vi "7HP v2.0 external control - EnFlo_Specific.vi"(6 "Datalog file path (full)":path, 7 "COM port":refnum<visa-resource-name>, 8 "Log data stream":bool, 9 "Set data rate (Hz)":u8(ring)=14 items=["1", "2", "4", "5", "8", "10", "16", "20", "25", "32", "40", "50", "64", "80", "100", "125", "160", "200", "250", "320", "400", "500", "625", "800", "1000"], 10 "N samples":u32=1000, 11 "Command":T2="D") -> (0 "Error":errorcluster, 1 "Returned data rate (Hz)":u16, 2 "Serial number":sgl, 3 "Data out":T3[](array[typedef]) {"Time stamp" format="%<%.6X\n%x>T"}, 4 "Rendezvous out":bool)   [LabVIEW 2021]
doc: "7HP test and configuration software.\nVersion 2.0\nSurrey Sensors Ltd.\n11/2023"
uses:
  ctls/7HP_Cmd (USB).ctl
  ctls/7HP_Data cluster.ctl
  Globals/Meas_global.vi
panel:
  in  "COM port 2":refnum<visa-resource-name>
  in  "Main":T1(tab)
  out "Subsystems ok":bool[](array[boolean])
  out "Pressure sensor values in range":bool[](array[boolean])
  out "Pressure sensor temperatures in range":bool[](array[boolean])
  out "Pressure sensor EEPROM checksums ok":bool[](array[boolean])
  out "P_raw_Azero":sgl[](array[numeric])
  out "n":u16
  out "Auto zero progBar":u16(slide) caption="Collecting samples, please maintain dP = 0" scale=0.0..1000.0
  in  "EEPROM array 2":u16[](array[numeric])
  in  "EEPROM array":sgl[](array[numeric]) format="%#.3f"
  out "EEPROM checksum ok":bool
  out "EEPROM checksum":u16 format="%04x"
  out "received":bool
  out "sent":bool
  out "Processed outputs":sgl[](array[numeric]) format="%#.2f"
  out "Frame errors":u32
  out "Checksum errors":u32
  in  "Stop Data":bool
  out "Rel. humidity (%)":sgl format="%#.2f"
  out "T_board (°C)":sgl format="%#.2f"
  out "T_external (°C)":sgl format="%#.2f"
  out "P_atmos (mbar)":sgl format="%#.2f"
  out "Checksum ok":bool
  out "Gyration vector (° / s)":sgl[](array[numeric]) format="%#.3f"
  out "Acceleration vector (g)":sgl[](array[numeric]) format="%#.3f"
  out "Pressures":sgl[][](graph)
  out "Stream enabled":bool
  out "Pitch (°)":sgl format="%.2f"
  out "Roll (°)":sgl format="%.2f"
  # "Paul Nathan 01/2024"
  # "Pressure sensor 0 EEPROM checksum okay"
  # "Pressure sensor 0 value in range"
  # "Pressure sensor 1 EEPROM checksum okay"
  # "Pressure sensor 1 value in range"
  # "Pressure sensor 2 EEPROM checksum okay"
  # "Pressure sensor 2 value in range"
  # "Pressure sensor 3 EEPROM checksum okay"
  # "Pressure sensor 3 value in range"
  # "Pressure sensor 4 EEPROM checksum okay"
  # "Pressure sensor 4 value in range"
  # "Pressure sensor 5 EEPROM checksum okay"
  # "Pressure sensor 5 value in range"
  # "Pressure sensor 6 EEPROM checksum okay"
  # "Pressure sensor 6 value in range"
  # "Pressure sensor 0 temperature in range"
  # "Environmental sensor present"
  # "Pressure sensor 1 temperature in range"
  # "Inertial sensor present"
  # "Pressure sensor 2 temperature in range"
  # "Accelerometer self test pass"
  # "Pressure sensor 3 temperature in range"
  # "Gyroscope self test pass"
  # "Pressure sensor 4 temperature in range"
  # "External thermistor value in range"
  # "Pressure sensor 5 temperature in range"
  # "MCU EEPROM checksum ok"
  # "Pressure sensor 6 temperature in range"
  # "%"
  # "P0 raw auto-zero"
  # "P1 raw auto-zero"
  # "P2 raw auto-zero"
  # "P3 raw auto-zero"
  # "P4 raw auto-zero"
  # "P5 raw auto-zero"
  # "P6 raw auto-zero"
  # "Power-up defaults"
  # "P0 raw auto-zero"
  # "Data rate (Hz)"
  # "P1 raw auto-zero"
  # "TTL streaming"
  # "P2 raw auto-zero"
  # "USB streaming"
  # "P3 raw auto-zero"
  # "TTL stream contains full data"
  # "P4 raw auto-zero"
  # "Accelerometer range mode"
  # "P5 raw auto-zero"
  # "Gyroscope range mode"
  # "P6 raw auto-zero"
  # "IMU rate mode"
  # "Atmospheric pressure offset (Pa)"
  # "HW trigger edge polarity"
  # "External thermistor temperature offset (°C)"
  # "Serial number"
  # "TTL baud rate (bps)"
  # "Accelerometer vector magnitude scale factor"
  # "Gyroscope x component offset (deg / s)"
  # "Gyroscope y component offset (deg / s)"
  # "Gyroscope z component offset (deg / s)"
  # "||U|| (m/s)"
  # "Pitch (deg)"
  # "Yaw (deg)"
  # "U (m/s)"
  # "V (m/s)"
  # "W (m/s)"
  # "w_x"
  # "w_y"
  # "w_z"
  # "a_x"
  # "a_y"
  # "a_z"
  # "||U|| (m/s)"
  # "Pitch (deg)"
  # "Yaw (deg)"
  # "U (m/s)"
  # "V (m/s)"
  # "W (m/s)"
  # "w_x"
  # "w_y"
  # "w_z"
  # "a_x"
  # "a_y"
  # "a_z"
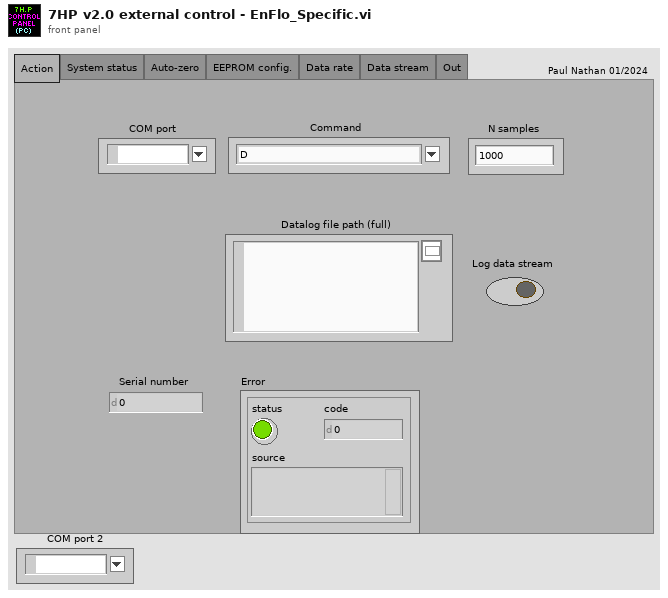
[diagram p1: front panel]
types:
  T1 = enum32{"Action", "System status", "Auto-zero", "EEPROM config.", "Data rate", "Data stream", "Out"}
  T2 = typedef "7HP_Cmd (USB).ctl" = string
  T3 = typedef "7HP_Data cluster.ctl" = cluster{"Time stamp":timestamp, "Pressures (Pa)":sgl[], "T_external (°C)":sgl, "P_atmos (mbar)":sgl, "T_board (°C)":sgl, "Rel. humidity (%)":sgl, "Acceleration vector (g)":sgl[], "Gyration vector (deg / s)":sgl[], "Processed outputs":sgl[]}
  T4 = enum16{"open", "replace", "create", "open or create", "replace or create", "replace or create with confirmation"}
  T5 = typedef "Rendezvous RefNum" = refnum<k1>
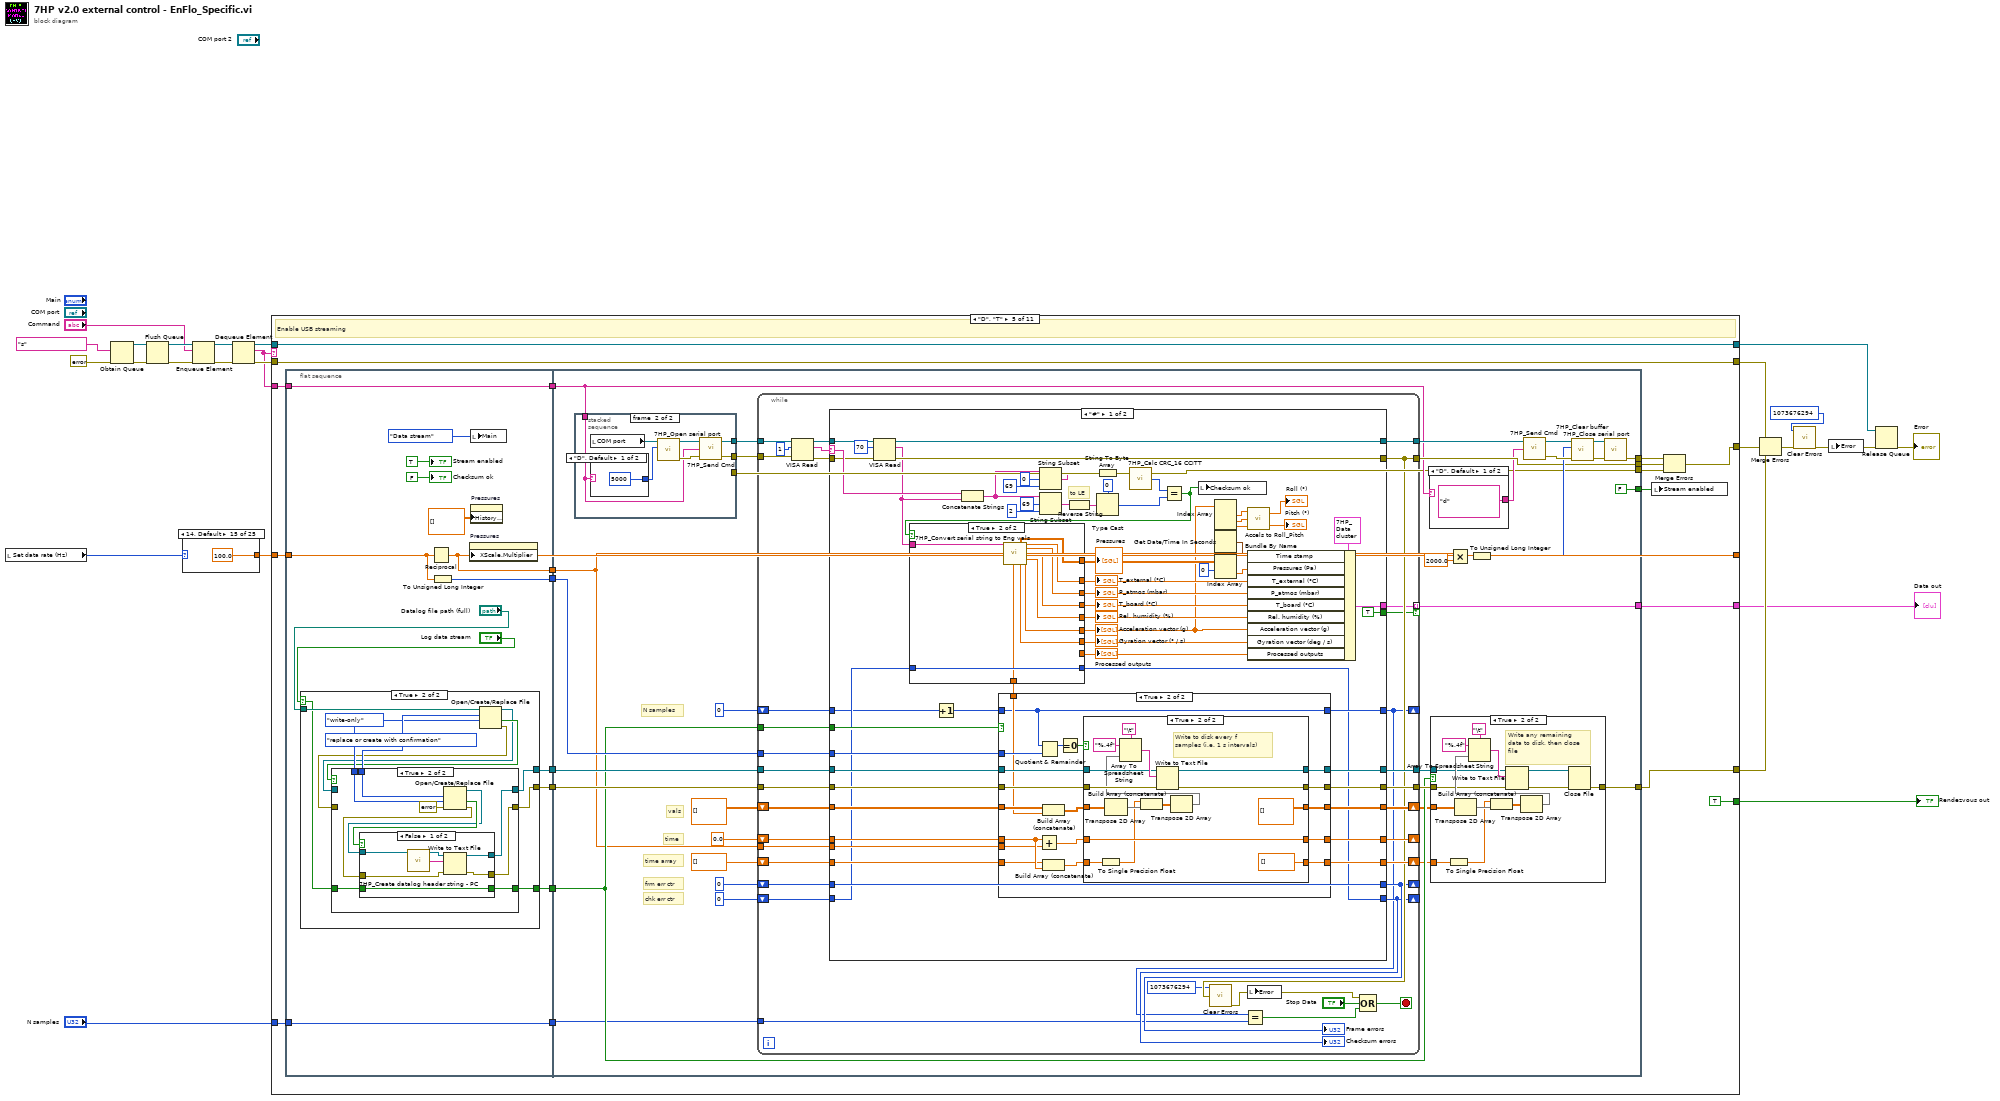
[diagram p0: block diagram]
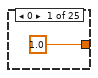
[diagram p2: hidden frame]
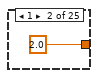
[diagram p3: hidden frame]
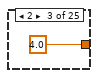
[diagram p4: hidden frame]
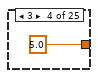
[diagram p5: hidden frame]
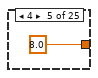
[diagram p6: hidden frame]
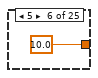
[diagram p7: hidden frame]
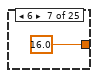
[diagram p8: hidden frame]
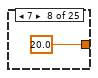
[diagram p9: hidden frame]
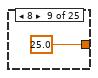
[diagram p10: hidden frame]
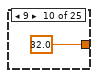
[diagram p11: hidden frame]
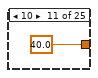
[diagram p12: hidden frame]
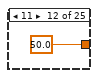
[diagram p13: hidden frame]
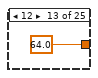
[diagram p14: hidden frame]
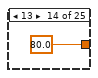
[diagram p15: hidden frame]
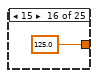
[diagram p16: hidden frame]
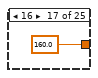
[diagram p17: hidden frame]
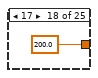
[diagram p18: hidden frame]
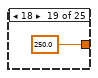
[diagram p19: hidden frame]
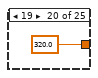
[diagram p20: hidden frame]
diagram:
  n1 = local read "Set data rate (Hz)"() -> (w4:u8)
  n2 = Obtain Queue(element data type=T2 "s" ("Combo Box"), error in (no error)=errorcluster {"status"=FALSE, "code"=0, "source"=""}) -> (queue out=w23:refnum<queue>, error out=w24:errorcluster)  [unwired: 3 in, 1 out]
  n3 = Flush Queue(queue=w23, error in (no error)=w24) -> (queue out=w19:refnum<queue>, error out=w20:errorcluster)  [unwired: 1 out]
  n4 = case shown="14, Default" w4 {
    tunnel: [1.0 2.0 4.0 5.0 8.0 10.0 16.0 20.0 25.0 32.0 40.0 50.0 64.0 80.0 100.0 125.0 160.0 200.0 250.0 320.0 400.0 500.0 625.0 800.0 1000.0] -> w5
    frame 0 {
    }
    frame 1 {
    }
    frame 2 {
    }
    frame 3 {
    }
    frame 4 {
    }
    frame 5 {
    }
    frame 6 {
    }
    frame 7 {
    }
    frame 8 {
    }
    frame 9 {
    }
    frame 10 {
    }
    frame 11 {
    }
    frame 12 {
    }
    frame 13 {
    }
    frame 14, Default {
    }
    frame 15 {
    }
    frame 16 {
    }
    frame 17 {
    }
    frame 18 {
    }
    frame 19 {
    }
    frame 20 {
    }
    frame 21 {
    }
    frame 22 {
    }
    frame 23 {
    }
    frame 24 {
    }
  }
  n5 = Enqueue Element(queue=w19, element="Command", error in (no error)=w20) -> (queue out=w18:refnum<queue>, error out=w17:errorcluster)  [unwired: 1 in, 1 out]
  n6 = Dequeue Element(queue=w18, error in (no error)=w17) -> (queue out=w15:refnum<queue>, element=w13:T2, error out=w14:errorcluster)  [unwired: 1 in, 1 out]
  n7 = case shown="\"D\", \"T\"" w13 {
    tunnel: [_ _ _ _ TRUE _ _ _ _ _ _] -> w1
    tunnel: w15 -> [w56 w95 w128 w190 w258 w547 w571 w627 w663 w685 w689]
    tunnel: [w56 w95 w128 w190 w258 w547 w571 w627 w663 w685 w689] -> w7
    tunnel: w14 -> [w55 w94 w127 w189 w257 w546 w572 w628 w662 w684 w688]
    tunnel: [w55 w94 w127 w189 w257 w546 w572 w628 w662 w684 w688] -> w12
    tunnel: w13 -> [w54 w93 w132 w196 w256 w549 w577 w633 w661 _ _]
    tunnel: [w52 w91 w130 w188 w244 w548 w570 w626 w659 errorcluster {"status"=FALSE, "code"=0, "source"=""} ("Error out") errorcluster {"status"=FALSE, "code"=0, "source"=""} ("Error out")] -> w11
    tunnel: [_ _ _ _ w254 _ _ _ _ _ _] -> w10
    tunnel: w5 -> [w51 w90 w129 w193 w247 w544 _ _ w658 w682 w686]
    tunnel: [w51 w90 w129 w193 w247 w544 w573 w629 w658 w682 w686] -> _
    tunnel: "N samples" -> [_ _ _ _ w242 _ _ _ _ _ _]
    tunnel: [_ _ _ _ w241 _ _ _ _ _ _] -> w2
    frame "S", "s" {
      # "Perform self-test and retrieve status bytes, Retrieve status bytes"
      n8 = flat-sequence {
        tunnel: w54 -> [w59]
        tunnel: [w59] -> w53
        tunnel: w53 -> [w65]
        tunnel: [w60] -> w52
        frame #0 {
          w58 = bool[] [] ("Pressure sensor EEPROM checksums ok")
          n9 = local write "Main"(T1."System status" ("Main")) -> ()
          "Pressure sensor EEPROM checksums ok" <- w58
          "Pressure sensor temperatures in range" <- w58
          "Pressure sensor values in range" <- w58
          "Subsystems ok" <- w58
        }
        frame #1 {
          w69 = 1 ("length (rest)")
          w77 = u8 0 ("byte count")
          n10 = local read "COM port"() -> (w66:refnum<visa-resource-name>)
          n11 = call "7HP_Open serial port.vi"("timeout (ms)"=u32 5000, "VISA resource name"=w66) -> ("Error out"=w87:errorcluster, "VISA resource name out"=w88:refnum<visa-resource-name>)  [unwired: 8 in]
          n12 = call "7HP_Send Cmd.vi"("Error In"=w87, "Operation"=w65, "Port"=w88) -> ("Error Out"=w85:errorcluster, "Port out"=w86:refnum<visa-resource-name>)  [unwired: 1 in]
          n13 = VISA Read(VISA resource name=w86, byte count=u32 4, error in (no error)=w85) -> (VISA resource name out=w83:refnum<visa-resource-name>, read buffer=w72:string, error out=w82:errorcluster)  [unwired: 1 out]
          n14 = call "7HP_Close serial port.vi"("Error in"=w82, "VISA resource name"=w83) -> ("Error out"=w60:errorcluster)  [unwired: 9 in]
          n15 = String Subset(string=w72, offset (0)=0, length (rest)=w69) -> (substring=w81:string)
          n16 = String Subset(string=w72, offset (0)=1, length (rest)=w69) -> (substring=w80:string)
          n17 = String Subset(string=w72, offset (0)=2 ("length (rest)"), length (rest)=w69) -> (substring=w79:string)
          n18 = String Subset(string=w72, offset (0)=3, length (rest)=w69) -> (substring=w78:string)
          n19 = Type Cast(type=w77, x=w81) -> (*(type *) &x=w76:u8)
          n20 = Type Cast(type=w77, x=w80) -> (*(type *) &x=w75:u8)
          n21 = Type Cast(type=w77, x=w79) -> (*(type *) &x=w74:u8)
          n22 = Type Cast(type=w77, x=w78) -> (*(type *) &x=w73:u8)
          n23 = Number To Boolean Array(number=w76) -> (Boolean array=w64:bool[])
          n24 = Number To Boolean Array(number=w75) -> (Boolean array=w63:bool[])
          n25 = Number To Boolean Array(number=w74) -> (Boolean array=w62:bool[])
          n26 = Number To Boolean Array(number=w73) -> (Boolean array=w61:bool[])
          n27 = local write "Pressure sensor EEPROM checksums ok"(w64) -> ()
          n28 = local write "Pressure sensor temperatures in range"(w63) -> ()
          n29 = local write "Pressure sensor values in range"(w62) -> ()
          n30 = local write "Subsystems ok"(w61) -> ()
        }
      }
    }
    frame "Z", "z" {
      # "Perform permanent auto-zero (write values to EEPROM), Perform temporary auto-zero"
      n31 = flat-sequence {
        tunnel: w93 -> [w99]
        tunnel: [w99] -> w92
        tunnel: w92 -> [w106]
        tunnel: [w102] -> w91
        frame #0 {
          n32 = local write "Main"(T1."Auto-zero" ("Main")) -> ()
          "P_raw_Azero" <- sgl[] [] ("P_raw_Azero")
          "Auto zero progBar" <- u16 0 ("Collecting samples, please maintain dP = 0")
        }
        frame #1 {
          n33 = local read "COM port"() -> (w107:refnum<visa-resource-name>)
          n34 = call "7HP_Open serial port.vi"("timeout (ms)"=u32 16000, "VISA resource name"=w107) -> ("Error out"=w113:errorcluster, "VISA resource name out"=w114:refnum<visa-resource-name>)  [unwired: 8 in]
          n35 = call "7HP_Send Cmd.vi"("Error In"=w113, "Operation"=w106, "Port"=w114) -> ("Error Out"=w111:errorcluster, "Port out"=w112:refnum<visa-resource-name>)  [unwired: 1 in]
          n36 = VISA Read(VISA resource name=w112, byte count=u32 28, error in (no error)=w111) -> (VISA resource name out=w109:refnum<visa-resource-name>, read buffer=w103:string, error out=w108:errorcluster)  [unwired: 1 out]
          n37 = for {
            N: 100 -> [_]
            shift-right: [w116] -> _
            shift-left: u16 0 -> [w117]
            n38 = Increment(x=w117) -> (x+1=w116:u16)
            "n" <- w116
            n39 = Wait (ms)(milliseconds to wait=u32 100) -> ()  [unwired: 1 out]
            n40 = local write "Auto zero progBar"(w116) -> ()
          }
          n41 = for {
            N: 7 -> [_]
            tunnel: [w120] -> w105 mode=indexing
            tunnel: w103 -> [w119]
            i -> [w126]
            w124 = 4 ("x")
            # "to BE"
            n42 = Multiply(x=w124, y=w126) -> (x*y=w125:i32)
            n43 = String Subset(string=w119, offset (0)=w125, length (rest)=w124) -> (substring=w123:string)
            n44 = Reverse String(1:w123) -> (0:w122:string)
            n45 = Type Cast(type=sgl 0.0 ("byte count"), x=w122) -> (*(type *) &x=w120:sgl)
          }
          n46 = call "7HP_Close serial port.vi"("Error in"=w108, "VISA resource name"=w109) -> ("Error out"=w102:errorcluster)  [unwired: 9 in]
          n47 = local write "P_raw_Azero"(w105) -> ()
        }
      }
    }
    frame "R" {
      # "Read all EEPROM values"
      n48 = flat-sequence {
        tunnel: w132 -> [w138]
        tunnel: [w138] -> w131
        tunnel: w131 -> [w170]
        tunnel: [w168] -> w130
        frame #0 {
          n49 = local write "EEPROM checksum ok"(FALSE ("Chk ok")) -> ()
          n50 = local write "EEPROM checksum"(u16 0 ("EEPROM checksum")) -> ()
          n51 = local write "EEPROM array"(sgl[] [] ("EEPROM array")) -> ()
          n52 = local write "EEPROM array 2"(u16[] [] ("EEPROM array 2")) -> ()
          n53 = local write "Main"(T1."EEPROM config." ("Main")) -> ()
        }
        frame #1 {
          # "to BE"
          # "to BE"
          n54 = local read "COM port"() -> (w171:refnum<visa-resource-name>)
          n55 = call "7HP_Open serial port.vi"("timeout (ms)"=u32 5000, "VISA resource name"=w171) -> ("Error out"=w177:errorcluster, "VISA resource name out"=w178:refnum<visa-resource-name>)  [unwired: 8 in]
          n56 = call "7HP_Send Cmd.vi"("Error In"=w177, "Operation"=w170, "Port"=w178) -> ("Error Out"=w175:errorcluster, "Port out"=w176:refnum<visa-resource-name>)  [unwired: 1 in]
          n57 = VISA Read(VISA resource name=w176, byte count=u32 71, error in (no error)=w175) -> (VISA resource name out=w173:refnum<visa-resource-name>, read buffer=w144:string, error out=w172:errorcluster)  [unwired: 1 out]
          n58 = call "7HP_Close serial port.vi"("Error in"=w172, "VISA resource name"=w173) -> ("Error out"=w168:errorcluster)  [unwired: 9 in]
          n59 = String Subset(string=w144, offset (0)=0, length (rest)=60 ("length (rest)")) -> (substring=w167:string)
          n60 = String Subset(string=w144, offset (0)=60, length (rest)=2 ("length (rest)")) -> (substring=w158:string)
          n61 = String Subset(string=w144, offset (0)=62, length (rest)=7 ("length (rest)")) -> (substring=w153:string)
          n62 = String Subset(string=w144, offset (0)=69, length (rest)=2 ("length (rest)")) -> (substring=w145:string)
          n63 = String Subset(string=w144, offset (0)=0, length (rest)=69 ("length (rest)")) -> (substring=w141:string)
          n64 = for {
            N: 15 -> [_]
            tunnel: [w183] -> w139 mode=indexing
            tunnel: w167 -> [w182]
            i -> [w187]
            w185 = 4 ("x")
            # "to BE"
            n65 = Multiply(x=w185, y=w187) -> (x*y=w186:i32)
            n66 = String Subset(string=w182, offset (0)=w186, length (rest)=w185) -> (substring=w181:string)
            n67 = Reverse String(1:w181) -> (0:w180:string)
            n68 = Type Cast(type=sgl 0.0 ("byte count"), x=w180) -> (*(type *) &x=w183:sgl)
          }
          n69 = Reverse String(1:w158) -> (0:w164:string)
          n70 = Reverse String(1:w145) -> (0:w149:string)
          n71 = String To Byte Array(string=w141) -> (unsigned byte array=w152:u8[])
          n72 = call "7HP_Calc CRC_16 CCITT.vi"("Data bytes"=w152) -> ("CRC_16-CCITT"=w151:u16)  [unwired: 1 in]
          n73 = Type Cast(type=u16 0 ("byte count"), x=w164) -> (*(type *) &x=w157:u16)
          n74 = Type Cast(type=u16 0 ("byte count"), x=w149) -> (*(type *) &x=w140:u16)
          n75 = String To Byte Array(string=w153) -> (unsigned byte array=w156:u8[])
          n76 = To Unsigned Word Integer(number=w156) -> (unsigned 16bit integer=w154:u16[])
          n77 = Equal?(x=w140, y=w151) -> (x = y?=w150:bool)
          n78 = Build Array (concatenate)(w157, w154) -> (w155:u16[])
          n79 = local write "EEPROM checksum ok"(w150) -> ()
          n80 = local write "EEPROM array"(w139) -> ()
          n81 = local write "EEPROM array 2"(w155) -> ()
          n82 = local write "EEPROM checksum"(w140) -> ()
        }
      }
    }
    frame "W" {
      # "Write all EEPROM values (including new checksum)"
      n83 = flat-sequence {
        tunnel: w196 -> [w206]
        tunnel: [w206] -> w195
        tunnel: ["EEPROM array"] -> w194
        tunnel: [w200] -> w192
        tunnel: [w201] -> w191
        tunnel: w195 -> [w228]
        tunnel: w194 -> [w223]
        tunnel: [w222] -> w188
        tunnel: w192 -> [w214]
        tunnel: w191 -> [w212]
        frame #0 {
          n84 = local write "Main"(T1."EEPROM config." ("Main")) -> ()
          n85 = Split 1D Array(array="EEPROM array 2", index=1) -> (first subarray=w203:u16[], second subarray=w202:u16[])
          n86 = Index Array(array=w203, index=0) -> (element=w200:u16)
          n87 = To Unsigned Byte Integer(number=w202) -> (unsigned 8bit integer=w201:u8[])
        }
        frame #1 {
          # "to LE"
          # "to LE"
          n88 = local read "COM port"() -> (w229:refnum<visa-resource-name>)
          n89 = for {
            N: 15 -> [_]
            tunnel: w223 -> [w235] mode=indexing
            shift-right: [w236] -> w218
            shift-left: "" -> [w237]
            # "to LE"
            n90 = Type Cast(type="", x=w235) -> (*(type *) &x=w234:string)
            n91 = Reverse String(1:w234) -> (0:w233:string)
            n92 = Concatenate Strings(w237, w233) -> (w236:string)
          }
          n93 = Type Cast(type="", x=w214) -> (*(type *) &x=w216:string)
          n94 = Reverse String(1:w216) -> (0:w213:string)
          n95 = Byte Array To String(unsigned byte array=w212) -> (string=w211:string)
          n96 = call "7HP_Open serial port.vi"("timeout (ms)"=u32 5000, "VISA resource name"=w229) -> ("Error out"=w230:errorcluster, "VISA resource name out"=w231:refnum<visa-resource-name>)  [unwired: 8 in]
          n97 = Concatenate Strings(w218, w213, w211) -> (w217:string)
          n98 = String To Byte Array(string=w217) -> (unsigned byte array=w210:u8[])
          n99 = call "7HP_Calc CRC_16 CCITT.vi"("Data bytes"=w210) -> ("CRC_16-CCITT"=w209:u16)  [unwired: 1 in]
          "EEPROM checksum" <- w209
          n100 = Type Cast(type="", x=w209) -> (*(type *) &x=w208:string)
          n101 = Reverse String(1:w208) -> (0:w207:string)
          n102 = Concatenate Strings(w217, w207) -> (w221:string)
          n103 = call "7HP_Send Cmd + Data.vi"("Error In"=w230, "Data"=w221, "Operation"=w228, "Port"=w231) -> ("Error Out"=w219:errorcluster, "Port out"=w220:refnum<visa-resource-name>)  [unwired: 1 in]
          n104 = call "7HP_Close serial port.vi"("Error in"=w219, "VISA resource name"=w220) -> ("Error out"=w222:errorcluster)  [unwired: 9 in]
          "EEPROM checksum ok" <- TRUE ("Chk ok")
        }
      }
    }
    frame "D", "T" {
      # "Enable USB streaming"
      n105 = flat-sequence {
        tunnel: w256 -> [w272]
        tunnel: [w272] -> w255
        tunnel: [w269] -> w253
        tunnel: [w268] -> w252
        tunnel: [w267] -> w251
        tunnel: w247 -> [w262]
        tunnel: [w261] -> w250
        tunnel: [w263] -> w249
        tunnel: [w260] -> w243
        tunnel: w242 -> [w260]
        tunnel: w255 -> [w314]
        tunnel: [w344] -> w245
        tunnel: [w343] -> w254
        tunnel: w253 -> [w340]
        tunnel: w252 -> [w339]
        tunnel: w251 -> [w341]
        tunnel: w250 -> [w323]
        tunnel: w249 -> [w333]
        tunnel: [FALSE] -> w248
        tunnel: [w318] -> w246
        tunnel: w243 -> [w315]
        tunnel: [w312] -> w241
        tunnel: [w311] -> w240
        frame #0 {
          n106 = case shown="True" "Log data stream" {
            selector: "Log data stream" -> [w273 w276]
            tunnel: "Datalog file path (full)" -> [_ w285]
            tunnel: [refnum<file> refnum ("refnum out") w282] -> w269
            tunnel: [errorcluster {"status"=FALSE, "code"=0, "source"=""} ("error out") w281] -> w268
            tunnel: [w273 w277] -> w263
            frame False {
            }
            frame True {
              w283 = enum16{"read/write", "read-only", "write-only"}."write-only" ("access (0:read/write)")
              w284 = T4."replace or create with confirmation" ("operation (0:open)")
              n107 = Open/Create/Replace File(file path (use dialog)=w285, operation (0:open)=w284, access (0:read/write)=w283) -> (refnum out=w278:refnum<file>, cancelled=w280:bool, error out=w279:errorcluster)  [unwired: 3 in]
              n108 = case shown="True" w280 {
                tunnel: w284 -> [_ w301]
                tunnel: w283 -> [_ w300]
                tunnel: w279 -> [w289 _]
                tunnel: [w287 w295] -> w282
                tunnel: [w288 w296] -> w281
                tunnel: w278 -> [w290 _]
                tunnel: [w286 w293] -> w277
                tunnel: w276 -> [w286 w292]
                frame False {
                  n109 = call "7HP_Create datalog header string - PC.vi"() -> ("Datalog header string"=w291:string)  [unwired: 1 in]
                  n110 = Write to Text File(file (use dialog)=w290, text=w291, error in=w289) -> (refnum out=w287:refnum<file>, error out=w288:errorcluster)  [unwired: 1 in, 1 out]
                }
                frame True {
                  n111 = Open/Create/Replace File(error in=errorcluster {"status"=FALSE, "code"=0, "source"=""}, operation (0:open)=w301, access (0:read/write)=w300) -> (refnum out=w298:refnum<file>, cancelled=w299:bool, error out=w297:errorcluster)  [unwired: 3 in]
                  n112 = case shown="False" w299 {
                    tunnel: w298 -> [w306 _]
                    tunnel: w297 -> [w305 _]
                    tunnel: [w304 errorcluster {"status"=FALSE, "code"=0, "source"=""} ("error out")] -> w296
                    tunnel: [w303 refnum<file> refnum ("t")] -> w295
                    tunnel: [w302 w308] -> w293
                    tunnel: w292 -> [w302 _]
                    frame False {
                      n113 = call "7HP_Create datalog header string - PC.vi"() -> ("Datalog header string"=w307:string)  [unwired: 1 in]
                      n114 = Write to Text File(file (use dialog)=w306, text=w307, error in=w305) -> (refnum out=w303:refnum<file>, error out=w304:errorcluster)  [unwired: 1 in, 1 out]
                    }
                    frame True {
                      w308 = FALSE ("Log data stream")
                      n115 = local write "Log data stream"(w308) -> ()
                    }
                  }
                }
              }
            }
          }
          n116 = Reciprocal(x=w262) -> (1/x=w261:dbl)
          n117 = To Unsigned Long Integer(number=w262) -> (unsigned 32bit integer=w267:u32)
          n118 = property on="Pressures" class="WFChart (strict)"("XScale.Multiplier"=w261) -> ()  [unwired: 2 in, 2 out]
          n119 = local write "Main"(T1."Data stream" ("Main")) -> ()
          n120 = property on="Pressures" class="WFChart (strict)"("History Data"=sgl[][] []) -> ()  [unwired: 2 in, 2 out]
          "Checksum ok" <- FALSE ("Checksum ok")
          "Stream enabled" <- TRUE ("Stream enabled")
        }
        frame #1 {
          # "N samples"
          # "chk err ctr"
          # "frm err ctr"
          # "vals"
          # "time"
          # "time array"
          n121 = stacked-sequence {
            tunnel: [_ w352] -> w332
            tunnel: [_ w350] -> w331
            tunnel: w314 -> [_ w348]
            tunnel: [w345 _] -> w311
            frame #0 {
              # "Wait here until all acq. devs. are ready."
              n122 = global read "Meas_global.vi" "Acquisition Rendezvous"() -> (w347:T5)
              n123 = call <vilib>:"Wait at Rendezvous.vi"("ms timeout (-1)"=60000, "rendezvous"=w347) -> ("error out"=w345:errorcluster)  [unwired: 3 in, 2 out]
            }
            frame #1 {
              n124 = local read "COM port"() -> (w354:refnum<visa-resource-name>)
              n125 = case shown="\"D\", Default" w348 {
                tunnel: [u32 5000 ("timeout (ms)") u32 15000 ("timeout (ms)")] -> w349
                frame "D", Default {
                }
                frame "T" {
                }
              }
              n126 = call "7HP_Open serial port.vi"("timeout (ms)"=w349, "VISA resource name"=w354) -> ("Error out"=w351:errorcluster, "VISA resource name out"=w353:refnum<visa-resource-name>)  [unwired: 8 in]
              n127 = call "7HP_Send Cmd.vi"("Error In"=w351, "Operation"=w348, "Port"=w353) -> ("Error Out"=w350:errorcluster, "Port out"=w352:refnum<visa-resource-name>)  [unwired: 1 in]
            }
          }
          n128 = while {
            tunnel: [w370] -> w318
            tunnel: w332 -> [w372]
            tunnel: [w389] -> w330
            shift-right: [w363] -> _
            shift-left: u32 0 -> [w386]
            tunnel: w341 -> [w385]
            tunnel: w340 -> [w384]
            tunnel: w339 -> [w383]
            tunnel: [w382] -> w338
            tunnel: [w381] -> w337
            shift-right: [w380] -> w320
            shift-left: sgl[][] [] -> [w379]
            shift-right: [w376] -> _
            shift-left: 0.0 ("Numeric") -> [w378]
            tunnel: w323 -> [w377]
            shift-right: [w374] -> w319
            shift-left: dbl[] [] -> [w375]
            tunnel: w333 -> [w373]
            tunnel: w331 -> [w371]
            shift-right: [w365] -> _
            shift-left: u32 0 -> [w367]
            shift-right: [w364] -> _
            shift-left: u32 0 -> [w366]
            tunnel: w315 -> [w362]
            tunnel: [w360] -> w312 mode=indexing if=w359
            stop <- w387 stop-if-true
            n129 = VISA Read(VISA resource name=w372, byte count=u32 1, error in (no error)=w371) -> (VISA resource name out=w391:refnum<visa-resource-name>, read buffer=w392:string, error out=w390:errorcluster)  [unwired: 1 out]
            n130 = case shown="\"#\"" w392 {
              selector: w392 -> [w435 _]
              tunnel: w391 -> [w421 w527]
              tunnel: [w451 w528] -> w370
              tunnel: w390 -> [w420 w528]
              tunnel: [w452 w527] -> w389
              tunnel: w386 -> [w414 w526]
              tunnel: [w450 w526] -> w363
              tunnel: w385 -> [w449 _]
              tunnel: w384 -> [w448 w525]
              tunnel: w383 -> [w447 w524]
              tunnel: [w446 w524] -> w382
              tunnel: [w445 w525] -> w381
              tunnel: [w444 w523] -> w380
              tunnel: w379 -> [w443 w523]
              tunnel: w378 -> [w442 w522]
              tunnel: w377 -> [w441 _]
              tunnel: [w440 w522] -> w376
              tunnel: w375 -> [w439 w521]
              tunnel: [w438 w521] -> w374
              tunnel: w373 -> [w437 _]
              tunnel: w367 -> [w436 w520]
              tunnel: w366 -> [w416 w519]
              tunnel: [w436 w518] -> w365
              tunnel: [w415 w519] -> w364
              tunnel: [w409 _] -> w360
              tunnel: [TRUE FALSE] -> w359
              frame "#" {
                # "to LE"
                n131 = VISA Read(VISA resource name=w421, byte count=u32 70, error in (no error)=w420) -> (VISA resource name out=w452:refnum<visa-resource-name>, read buffer=w419:string, error out=w451:errorcluster)  [unwired: 1 out]
                n132 = Increment(x=w414) -> (x+1=w413:u32)
                n133 = Concatenate Strings(w435, w419) -> (w423:string)
                n134 = String Subset(string=w423, offset (0)=0, length (rest)=69 ("length (rest)")) -> (substring=w422:string)
                n135 = String Subset(string=w423, offset (0)=69, length (rest)=2 ("length (rest)")) -> (substring=w429:string)
                n136 = Reverse String(1:w429) -> (0:w428:string)
                n137 = String To Byte Array(string=w422) -> (unsigned byte array=w433:u8[])
                n138 = Type Cast(type=u16 0 ("length (rest)"), x=w428) -> (*(type *) &x=w427:u16)
                n139 = call "7HP_Calc CRC_16 CCITT.vi"("Data bytes"=w433) -> ("CRC_16-CCITT"=w426:u16)  [unwired: 1 in]
                n140 = Equal?(x=w426, y=w427) -> (x = y?=w417:bool)
                n141 = case shown="True" w417 {
                  tunnel: w419 -> [_ w470]
                  tunnel: [w459 w469] -> w411
                  tunnel: [w455 w468] -> w405
                  tunnel: [w455 w467] -> w404
                  tunnel: [w455 w466] -> w403
                  tunnel: [w455 w465] -> w402
                  tunnel: [w454 w464] -> w394
                  tunnel: [w454 w463] -> w401
                  tunnel: [w456 w461] -> w418
                  tunnel: w416 -> [w458 w462]
                  tunnel: [w457 w462] -> w415
                  tunnel: [sgl[] [nan, nan, nan, nan, nan, nan] _] -> w400
                  frame False {
                    w460 = sgl[] [nan, nan, nan, nan, nan, nan, nan]
                    w455 = sgl nan
                    w454 = sgl[] [nan, nan, nan]
                    n142 = Increment(x=w458) -> (x+1=w457:u32)
                    n143 = Build Array (concatenate)(w460, w455, w455, w455, w455, w454, w454) -> (w456:sgl[])
                    n144 = Build Array(w460) -> (w459:sgl[][])
                  }
                  frame True {
                    n145 = call "7HP_Convert serial string to Eng vals.vi"("Serial buffer string (excluding FrameChar)"=w470) -> ("All vals"=w461:sgl[], "Pressures"=w469:sgl[][], "Gyration vector (deg / s)"=w463:sgl[], "External thermistor temperature (deg C)"=w468:sgl, "Atmospheric pressure (mbar)"=w467:sgl, "Env. sensor die temperature (deg C)"=w466:sgl, "Relative humidity (%)"=w465:sgl, "Acceleration vector (g)"=w464:sgl[])  [unwired: 11 in]
                  }
                }
                "Pressures" <- w411
                "Acceleration vector (g)" <- w394
                "Gyration vector (° / s)" <- w401
                "P_atmos (mbar)" <- w404
                "T_external (°C)" <- w405
                "T_board (°C)" <- w403
                "Rel. humidity (%)" <- w402
                "Processed outputs" <- w400
                n146 = case shown="True" w437 {
                  tunnel: w413 -> [w476 w477]
                  tunnel: [w476 w477] -> w450
                  tunnel: w449 -> [_ w495]
                  tunnel: w418 -> [_ w481]
                  tunnel: w448 -> [w474 w492]
                  tunnel: w447 -> [w475 w491]
                  tunnel: [w475 w490] -> w446
                  tunnel: [w474 w489] -> w445
                  tunnel: w443 -> [w473 w482]
                  tunnel: [w473 w488] -> w444
                  tunnel: w442 -> [w472 w485]
                  tunnel: w441 -> [_ w484]
                  tunnel: [w472 w487] -> w440
                  tunnel: w439 -> [w471 w483]
                  tunnel: [w471 w486] -> w438
                  frame False {
                  }
                  frame True {
                    n147 = Add(x=w485, y=w484) -> (x+y=w480:dbl)
                    n148 = Quotient & Remainder(x=w477, y=w495) -> (x-y*floor(x/y)=w494:u32)  [unwired: 1 out]
                    n149 = Build Array (concatenate)(w482, w481) -> (w478:sgl[][])
                    n150 = Build Array (concatenate)(w483, w485) -> (w479:dbl[])
                    n151 = Equal To 0?(x=w494) -> (x = 0?=w493:bool)
                    n152 = case shown="True" w493 {
                      tunnel: w492 -> [w499 w513]
                      tunnel: w491 -> [w500 w512]
                      tunnel: [w500 w511] -> w490
                      tunnel: [w499 w510] -> w489
                      tunnel: w478 -> [w497 w505]
                      tunnel: [w497 sgl[][] []] -> w488
                      tunnel: w480 -> [w498 w508]
                      tunnel: [w498 w508] -> w487
                      tunnel: w479 -> [w496 w507]
                      tunnel: [w496 dbl[] []] -> w486
                      frame False {
                      }
                      frame True {
                        # "Write to disk every f samples (i.e. 1 s intervals)"
                        n153 = To Single Precision Float(number=w507) -> (single precision float=w501:sgl[])
                        n154 = Transpose 2D Array(2D array=w505) -> (transposed array=w504:sgl[][])
                        n155 = Build Array (concatenate)(w501, w504) -> (w503:sgl[][])
                        n156 = Transpose 2D Array(2D array=w503) -> (transposed array=w502:sgl[][])
                        n157 = Array To Spreadsheet String(delimiter (Tab)="\t", array=w502, 3:"%.4f" ("format string")) -> (spreadsheet string=w516:string)
                        n158 = Write to Text File(file (use dialog)=w513, text=w516, error in=w512) -> (refnum out=w510:refnum<file>, error out=w511:errorcluster)  [unwired: 1 in, 1 out]
                      }
                    }
                  }
                }
                n159 = local write "Checksum ok"(w417) -> ()
                n160 = Index Array(array=w394) -> (element #1=w399:sgl, element #2=w398:sgl, element #3=w397:sgl)  [unwired: 3 in]
                n161 = Get Date/Time In Seconds() -> (seconds since 1Jan1904=w407:timestamp)
                n162 = Index Array(array=w411, index (row)=0) -> (element=w406:sgl[])  [unwired: 1 in]
                n163 = call "Accels to Roll_Pitch.vi"("az"=w397, "ay"=w398, "ax"=w399) -> ("Pitch (deg)"=→"Pitch (°)":sgl, "Roll (deg)"=→"Roll (°)":sgl)
                n164 = Bundle By Name(cluster=T3 {"Time stamp"=timestamp(0 s since 1904-01-01), "Pressures (Pa)"=[], "T_external (°C)"=0.0, "P_atmos (mbar)"=0.0, "T_board (°C)"=0.0, "Rel. humidity (%)"=0.0, "Acceleration vector (g)"=[], "Gyration vector (deg / s)"=[], "Processed outputs"=[]} ("Data cluster 7HP"), "Time stamp"=w407, "Pressures (Pa)"=w406, "T_external (°C)"=w405, "P_atmos (mbar)"=w404, "T_board (°C)"=w403, "Rel. humidity (%)"=w402, "Acceleration vector (g)"=w394, "Gyration vector (deg / s)"=w401, "Processed outputs"=w400) -> (w409:T3)
              }
              frame Default {
                # "Frame error"
                n165 = Increment(x=w520) -> (x+1=w518:u32)
              }
            }
            "Checksum errors" <- w364
            "Frame errors" <- w365
            n166 = call <vilib>:"Clear Errors.vi"("error in (no error)"=w370, "specific error code to clear (0: all)"=1073676294) -> ("error out"=w369:errorcluster)  [unwired: 4 in, 1 out]
            n167 = Equal?(x=w363, y=w362) -> (x = y?=w361:bool)
            n168 = local write "Error"(w369) -> ()
            n169 = Compound Arithmetic op=OR(w369, "Stop Data", w361) -> (w387:bool)
          }
          n170 = case shown="\"D\", Default" w314 {
            tunnel: [T2 "d" ("Combo Box") T2 "t" ("Combo Box")] -> w313
            frame "D", Default {
            }
            frame "T" {
            }
          }
          n171 = case shown="True" w333 {
            tunnel: [w529 w543] -> w343
            tunnel: w338 -> [w529 w535]
            tunnel: w337 -> [_ w536]
            tunnel: w320 -> [_ w534]
            tunnel: w319 -> [_ w533]
            frame False {
            }
            frame True {
              # "Write any remaining data to disk, then close file"
              n172 = To Single Precision Float(number=w533) -> (single precision float=w530:sgl[])
              n173 = Transpose 2D Array(2D array=w534) -> (transposed array=w540:sgl[][])
              n174 = Build Array (concatenate)(w530, w540) -> (w541:sgl[][])
              n175 = Transpose 2D Array(2D array=w541) -> (transposed array=w542:sgl[][])
              n176 = Array To Spreadsheet String(delimiter (Tab)="\t", array=w542, 3:"%.4f" ("format string")) -> (spreadsheet string=w537:string)
              n177 = Write to Text File(file (use dialog)=w536, text=w537, error in=w535) -> (refnum out=w532:refnum<file>, error out=w531:errorcluster)  [unwired: 1 in, 1 out]
              n178 = Close File(refnum=w532, error in=w531) -> (error out=w543:errorcluster)  [unwired: 1 out]
            }
          }
          n179 = Multiply(x=w323, y=2000.0) -> (x*y=w324:dbl)
          n180 = To Unsigned Long Integer(number=w324) -> (unsigned 32bit integer=w321:u32)
          n181 = call "7HP_Send Cmd.vi"("Operation"=w313, "Port"=w330) -> ("Error Out"=w327:errorcluster, "Port out"=w328:refnum<visa-resource-name>)  [unwired: 2 in]
          n182 = call "7HP_Clear buffer.vi"("Error in"=w327, "dt for timeout (ms)"=w321, "VISA resource name in"=w328) -> ("Error out"=w325:errorcluster, "VISA resource name out"=w326:refnum<visa-resource-name>)  [unwired: 3 in]
          n183 = call "7HP_Close serial port.vi"("Error in"=w325, "VISA resource name"=w326) -> ("Error out"=w344:errorcluster)  [unwired: 9 in]
        }
      }
      n184 = local write "Stream enabled"(w248) -> ()
      n185 = Merge Errors(w245, w246, w240) -> (w244:errorcluster)
    }
    frame "d", "t" {
      # "Disable USB streaming"
      n186 = flat-sequence {
        tunnel: [w557] -> w550
        tunnel: w549 -> [w557]
        tunnel: w544 -> [w556]
        tunnel: [w551] -> w545
        tunnel: w550 -> [w565]
        tunnel: [w564] -> w548
        tunnel: w545 -> [w559]
        frame #0 {
          n187 = Reciprocal(x=w556) -> (1/x=w555:dbl)
          n188 = disable-structure shown="Disabled" {
            frame Disabled {
              n189 = local write "Main"(T1."Data stream" ("Main")) -> ()
            }
            frame Enabled {
            }
          }
          n190 = To Single Precision Float(number=w555) -> (single precision float=w552:sgl)
          n191 = Multiply(x=w552, y=sgl 2000.0) -> (x*y=w553:sgl)
          n192 = To Unsigned Long Integer(number=w553) -> (unsigned 32bit integer=w551:u32)
        }
        frame #1 {
          n193 = local read "COM port"() -> (w566:refnum<visa-resource-name>)
          n194 = call "7HP_Open serial port.vi"("timeout (ms)"=u32 5000, "VISA resource name"=w566) -> ("Error out"=w567:errorcluster, "VISA resource name out"=w568:refnum<visa-resource-name>)  [unwired: 8 in]
          n195 = call "7HP_Send Cmd.vi"("Error In"=w567, "Operation"=w565, "Port"=w568) -> ("Error Out"=w563:errorcluster, "Port out"=w561:refnum<visa-resource-name>)  [unwired: 1 in]
          n196 = call "7HP_Clear buffer.vi"("Error in"=w563, "dt for timeout (ms)"=w559, "VISA resource name in"=w561) -> ("Error out"=w562:errorcluster, "VISA resource name out"=w560:refnum<visa-resource-name>)  [unwired: 3 in]
          n197 = call "7HP_Close serial port.vi"("Error in"=w562, "VISA resource name"=w560) -> ("Error out"=w564:errorcluster)  [unwired: 9 in]
        }
      }
    }
    frame "F" {
      # "Set data rate"
      n198 = flat-sequence {
        tunnel: w577 -> [w581]
        tunnel: [w581] -> w576
        tunnel: w576 -> [w586]
        tunnel: [w585] -> w575
        tunnel: [w584] -> w574
        tunnel: [w624] -> w573
        tunnel: w575 -> [w624]
        tunnel: w574 -> [w622]
        tunnel: [w622] -> w570
        frame #0 {
          n199 = local write "Returned data rate (Hz)"(u16 0 ("Returned data rate (Hz)")) -> ()
          n200 = local write "received"(FALSE ("sent")) -> ()
          n201 = local write "Main"(T1."Data rate" ("Main")) -> ()
          n202 = local write "sent"(FALSE ("sent")) -> ()
        }
        frame #1 {
          # "to LE"
          n203 = case shown="14, Default" "Set data rate (Hz)" {
            tunnel: [1.0 2.0 4.0 5.0 8.0 10.0 16.0 20.0 25.0 32.0 40.0 50.0 64.0 80.0 100.0 125.0 160.0 200.0 250.0 320.0 400.0 500.0 625.0 800.0 1000.0] -> w585
            frame 0 {
            }
            frame 1 {
            }
            frame 2 {
            }
            frame 3 {
            }
            frame 4 {
            }
            frame 5 {
            }
            frame 6 {
            }
            frame 7 {
            }
            frame 8 {
            }
            frame 9 {
            }
            frame 10 {
            }
            frame 11 {
            }
            frame 12 {
            }
            frame 13 {
            }
            frame 14, Default {
            }
            frame 15 {
            }
            frame 16 {
            }
            frame 17 {
            }
            frame 18 {
            }
            frame 19 {
            }
            frame 20 {
            }
            frame 21 {
            }
            frame 22 {
            }
            frame 23 {
            }
            frame 24 {
            }
          }
          n204 = local read "COM port"() -> (w589:refnum<visa-resource-name>)
          n205 = To Unsigned Word Integer(number=w585) -> (unsigned 16bit integer=w594:u16)
          n206 = Type Cast(type="", x=w594) -> (*(type *) &x=w596:string)
          n207 = call "7HP_Open serial port.vi"("timeout (ms)"=u32 5000, "VISA resource name"=w589) -> ("Error out"=w590:errorcluster, "VISA resource name out"=w591:refnum<visa-resource-name>)  [unwired: 8 in]
          n208 = Reverse String(1:w596) -> (0:w583:string)
          n209 = call "7HP_Send Cmd + Data.vi"("Error In"=w590, "Data"=w583, "Operation"=w586, "Port"=w591) -> ("Error Out"=w587:errorcluster, "Port out"=w588:refnum<visa-resource-name>)  [unwired: 1 in]
          n210 = call "7HP_Close serial port.vi"("Error in"=w587, "VISA resource name"=w588) -> ("Error out"=w584:errorcluster)  [unwired: 9 in]
        }
        frame #2 {
          n211 = Unbundle By Name(w622) -> ("status"=w623:bool)
          n212 = Not(x=w623) -> (.not. x?=→"sent":bool)
        }
      }
    }
    frame "f" {
      # "Get data rate"
      n213 = flat-sequence {
        tunnel: w633 -> [w637]
        tunnel: [w637] -> w632
        tunnel: w632 -> [w646]
        tunnel: [w649] -> w631
        tunnel: [w651] -> w630
        tunnel: [w657] -> w629
        tunnel: w631 -> [w657]
        tunnel: w630 -> [w655]
        tunnel: [w655] -> w626
        frame #0 {
          n214 = local write "received"(FALSE ("sent")) -> ()
          n215 = local write "Main"(T1."Data rate" ("Main")) -> ()
          n216 = local write "sent"(FALSE ("sent")) -> ()
        }
        frame #1 {
          # "to BE"
          n217 = local read "COM port"() -> (w652:refnum<visa-resource-name>)
          n218 = call "7HP_Open serial port.vi"("timeout (ms)"=u32 5000, "VISA resource name"=w652) -> ("Error out"=w647:errorcluster, "VISA resource name out"=w648:refnum<visa-resource-name>)  [unwired: 8 in]
          n219 = call "7HP_Send Cmd.vi"("Error In"=w647, "Operation"=w646, "Port"=w648) -> ("Error Out"=w644:errorcluster, "Port out"=w643:refnum<visa-resource-name>)  [unwired: 1 in]
          n220 = VISA Read(VISA resource name=w643, byte count=u32 2, error in (no error)=w644) -> (VISA resource name out=w641:refnum<visa-resource-name>, read buffer=w640:string, error out=w642:errorcluster)  [unwired: 1 out]
          n221 = Reverse String(1:w640) -> (0:w650:string)
          n222 = call "7HP_Close serial port.vi"("Error in"=w642, "VISA resource name"=w641) -> ("Error out"=w651:errorcluster)  [unwired: 9 in]
          n223 = Type Cast(type=u16 0 ("byte count"), x=w650) -> (*(type *) &x=w638:u16)
          "Returned data rate (Hz)" <- w638
          n224 = To Double Precision Float(number=w638) -> (double precision float=w649:dbl)
        }
        frame #2 {
          n225 = Unbundle By Name(w655) -> ("status"=w656:bool)
          n226 = Not(x=w656) -> (.not. x?=→"received":bool)
        }
      }
    }
    frame "N" {
      # "Get serial number"
      n227 = flat-sequence {
        tunnel: w661 -> [w666]
        tunnel: [w666] -> w660
        tunnel: w660 -> [w672]
        tunnel: [w671] -> w659
        frame #0 {
          n228 = local write "Main"(T1."Action" ("Main")) -> ()
          "Serial number" <- sgl 0.0 ("Numeric")
        }
        frame #1 {
          # "to BE"
          n229 = local read "COM port"() -> (w673:refnum<visa-resource-name>)
          n230 = call "7HP_Open serial port.vi"("timeout (ms)"=u32 5000, "VISA resource name"=w673) -> ("Error out"=w679:errorcluster, "VISA resource name out"=w680:refnum<visa-resource-name>)  [unwired: 8 in]
          n231 = call "7HP_Send Cmd.vi"("Error In"=w679, "Operation"=w672, "Port"=w680) -> ("Error Out"=w677:errorcluster, "Port out"=w678:refnum<visa-resource-name>)  [unwired: 1 in]
          n232 = VISA Read(VISA resource name=w678, byte count=u32 4, error in (no error)=w677) -> (VISA resource name out=w675:refnum<visa-resource-name>, read buffer=w668:string, error out=w674:errorcluster)  [unwired: 1 out]
          n233 = call "7HP_Close serial port.vi"("Error in"=w674, "VISA resource name"=w675) -> ("Error out"=w671:errorcluster)  [unwired: 9 in]
          n234 = Reverse String(1:w668) -> (0:w669:string)
          n235 = Type Cast(type=sgl 0.0 ("byte count"), x=w669) -> (*(type *) &x=w667:sgl)
          n236 = local write "Serial number"(w667) -> ()
        }
      }
    }
    frame "X" {
      # "Exit"
    }
    frame Default {
    }
  }
  "Data out" <- w2
  "Rendezvous out" <- w1
  n237 = Merge Errors(w12, w11, w10) -> (w9:errorcluster)
  n238 = call <vilib>:"Clear Errors.vi"("error in (no error)"=w9, "specific error code to clear (0: all)"=1073676294) -> ("error out"=w6:errorcluster)  [unwired: 4 in, 1 out]
  n239 = local write "Error"(w6) -> ()
  n240 = Release Queue(queue=w7, error in (no error)=w6) -> (error out=→"Error":errorcluster)  [unwired: 1 in, 2 out]
